vi "PCAN_identification.vi"(8 "error in (no error)":errorcluster, 10 "PCAN_ID":string, 11 "module path":path) -> (0 "error out":errorcluster, 3 "return value":i32 format="%.0x")   [LabVIEW 2024, in "PCANusb_DTU.lvlib"]
uses:
  PCANusb_DTU.lvlib
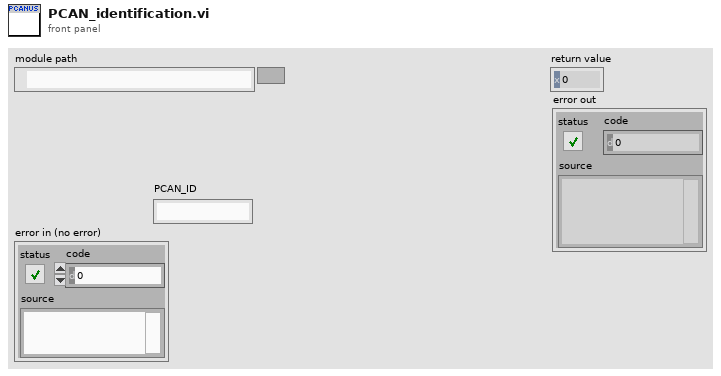
[diagram p1: front panel]
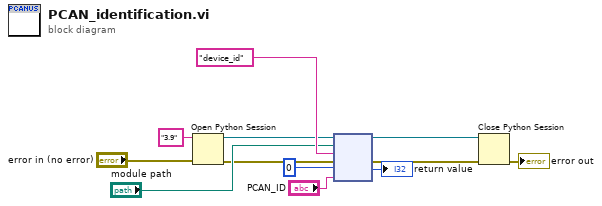
[diagram p0: block diagram]
diagram:
  n1 = Open Python Session(python version="3.9" ("Python version"), 3:"error in (no error)") -> (session out=w10:refnum<k35>, error out=w5:errorcluster)  [unwired: 1 in]
  n2 = node(w10, "module path", "device_id", w5, 0, "PCAN_ID") -> (w2:refnum<k35>, w3:errorcluster, →"return value":i32)  [unwired: 1 in, 2 out]
  n3 = Close Python Session(session in=w2, error in=w3) -> (11:→"error out":errorcluster)
